vi "Parsing Error.vi"(6 "initial string":string, 7 "JSON":string, 8 "error in (no error)":errorcluster, 9 "Offset past match":i32=-1, 10 "Value start":i32=-1, 11 "State":T1) -> (0 "error out":errorcluster)   [LabVIEW 2017, in "JSONtext.lvlib"]
uses:
  JSONtext.lvlib
  Parsing State.ctl
  <vilib>/JDP Science/JDP Science Common Utilities/JDP Utility.lvlib
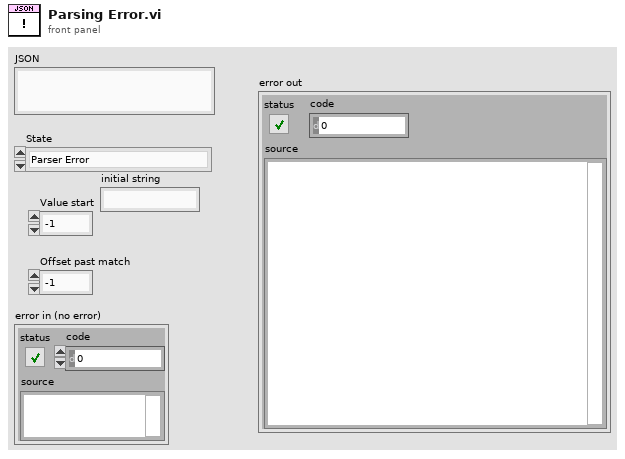
[diagram p1: front panel]
types:
  T1 = typedef "JSONtext.lvlib/Parsing State.ctl" = enum16{"Parser Error", "Object", "Array", "String", "Number/Other", "Leading Whitespace", "Object end", "Array end", "Value end"}
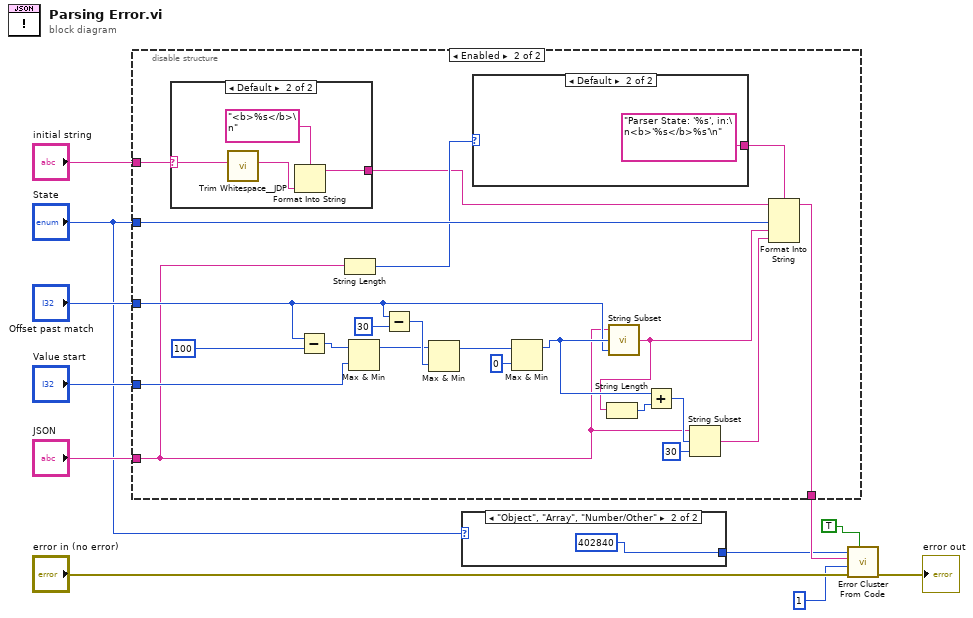
[diagram p0: block diagram]
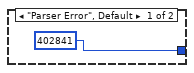
[diagram p2: hidden frame]
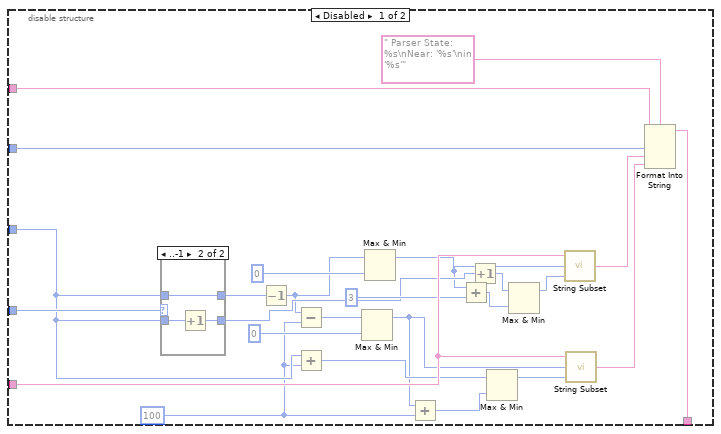
[diagram p3: hidden frame]
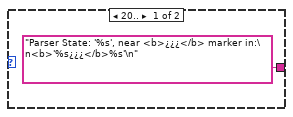
[diagram p6: hidden frame]
diagram:
  n1 = disable-structure shown="Enabled" {
    disable-tunnel: "State" -> [w36 w63]
    disable-tunnel: [w35 w62] -> w11
    disable-tunnel: "JSON" -> [w32 w44]
    disable-tunnel: "Value start" -> [w28 w58]
    disable-tunnel: "Offset past match" -> [w27 w47]
    disable-tunnel: "initial string" -> [w26 w43]
    frame Disabled {
      w23 = 100 ("y")
      n2 = case shown="..-1" w28 {
        selector: w28 -> [w38 _]
        tunnel: [w38 w41] -> w20
        tunnel: w27 -> [_ w41]
        tunnel: w27 -> [w37 w39]
        tunnel: [w37 w40] -> w17
        frame Default {
        }
        frame ..-1 {
          n3 = Increment(x=w39) -> (x+1=w40:i32)
        }
      }
      n4 = Decrement(x=w20) -> (x-1=w14:i32)
      n5 = Subtract(x=w14, y=w23) -> (x-y=w31:i32)
      n6 = Add(x=w27, y=w23) -> (x+y=w29:i32)
      n7 = Max & Min(x=w31, y=0) -> (max(x,y)=w24:i32)  [unwired: 1 out]
      n8 = Max & Min(x=w14, y=0) -> (max(x,y)=w13:i32)  [unwired: 1 out]
      n9 = Add(x=w24, y=w23) -> (x+y=w21:i32)
      n10 = Add(x=w13, y=3) -> (x+y=w18:i32)
      n11 = Increment(x=w17) -> (x+1=w12:i32)
      n12 = Max & Min(x=w29, y=w21) -> (max(x,y)=w22:i32)  [unwired: 1 out]
      n13 = Max & Min(x=w12, y=w18) -> (max(x,y)=w16:i32)  [unwired: 1 out]
      n14 = call "String Subset.vi"("Offset past End"=w16, "Start offset"=w13, "JSON"=w32) -> ("substring"=w34:string)  [unwired: 2 in]
      n15 = call "String Subset.vi"("Offset past End"=w22, "Start offset"=w24, "JSON"=w32) -> ("substring"=w30:string)  [unwired: 2 in]
      n16 = Format Into String(format string=" Parser State: %s\nNear: '%s'\nin '%s'", initial string=w26, w36, w34, w30) -> (resulting string=w35:string)  [unwired: 1 in, 1 out]
    }
    frame Enabled {
      n17 = case shown="Default" w43 {
        selector: w43 -> [_ w67]
        tunnel: [_ w66] -> w42
        frame "" {
        }
        frame Default {
          n18 = call <vilib>:"Trim Whitespace__JDP.vi"("String in"=w67) -> ("String out"=w64:string)  [unwired: 6 in]
          n19 = Format Into String(format string="<b>%s</b>\n", w64) -> (resulting string=w66:string)  [unwired: 2 in, 1 out]
        }
      }
      n20 = Subtract(x=w47, y=100) -> (x-y=w59:i32)
      n21 = String Length(string=w44) -> (length=w45:i32)
      n22 = Max & Min(x=w59, y=w58) -> (max(x,y)=w49:i32)  [unwired: 1 out]
      n23 = Subtract(x=w47, y=30) -> (x-y=w50:i32)
      n24 = Max & Min(x=w49, y=w50) -> (max(x,y)=w48:i32)  [unwired: 1 out]
      n25 = case shown="Default" w45 {
        tunnel: ["Parser State: '%s', near <b>¿¿¿</b> marker in:\n<b>'%s¿¿¿</b>%s'\n" ("format string") "Parser State: '%s', in:\n<b>'%s</b>%s'\n" ("format string")] -> w46
        frame 20.. {
        }
        frame Default {
        }
      }
      n26 = Max & Min(x=w48, y=0) -> (max(x,y)=w56:i32)  [unwired: 1 out]
      n27 = call "String Subset.vi"("Offset past End"=w47, "Start offset"=w56, "JSON"=w44) -> ("substring"=w54:string)  [unwired: 2 in]
      n28 = String Length(string=w54) -> (length=w55:i32)
      n29 = Add(x=w56, y=w55) -> (x+y=w53:i32)
      n30 = String Subset(string=w44, offset (0)=w53, length (rest)=30 ("Offset past End")) -> (substring=w61:string)
      n31 = Format Into String(format string=w46, initial string=w42, w63, w54, w61) -> (resulting string=w62:string)  [unwired: 1 in, 1 out]
    }
  }
  n32 = case shown="\"Object\", \"Array\", \"Number/Other\"" "State" {
    tunnel: [402841 ("error code (0)") 402840 ("error code (0)")] -> w1
    frame "Parser Error", Default {
    }
    frame "Object", "Array", "Number/Other" {
    }
  }
  n33 = call "Error Cluster From Code.vi"("show call chain? (True)"=TRUE ("show call chain? (False)"), "error in (no error)"="error in (no error)", "Call Depth"=1, "error message (\"\")"=w11, "error code (402840+)"=w1) -> ("error out"=→"error out":errorcluster)  [unwired: 4 in]
